vi "Configure Sequencer List ARB Cycles.vi"(7 "ARB Cycles (1)":i32=1, 8 "error in (no error)":errorcluster, 9 "Index (0)":i32, 10 "Instance (1)":i32=1, 11 "VISA resource name":refnum<visa-resource-name>) -> (0 "error out":errorcluster, 3 "VISA resource name out":refnum<visa-resource-name>)   [LabVIEW 2020, in "Rohde&Schwarz CMXP GPRF.lvlib"]
doc: "Defines the number of ARB cycles for the sequencer list entry with the selected Index.\n\nAttribute:\nRSCMXPGPRF_ATTR_SEQUENCER_LIST_ARB_CYCLES\n\nRemote-control command:\nSOURce:GPRF:GEN<i>:SEQuencer:LIST:ACYCles"
uses:
  <instrlib>/Rohde&Schwarz CMXP GPRF/Rohde&Schwarz CMXP GPRF.lvlib
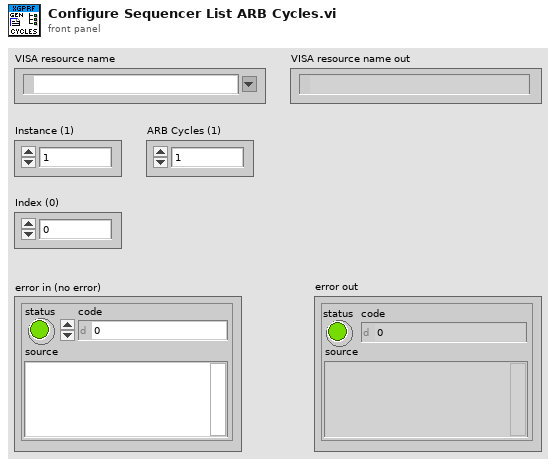
[diagram p1: front panel]
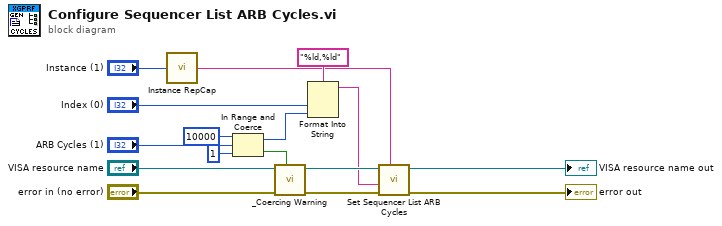
[diagram p0: block diagram]
diagram:
  n1 = call <instrlib>:"Instance RepCap.vi"("Instance in"="Instance (1)") -> ("Instance out"=w3:string)
  n2 = In Range and Coerce(upper limit=10000, x="ARB Cycles (1)", lower limit=1) -> (coerced(x)=w2:i32, In Range?=w10:bool)
  n3 = call <instrlib>:"_Coercing Warning.vi"("In Range?"=w10, "error in (no error)"="error in (no error)", "VISA resource name"="VISA resource name") -> ("error out"=w7:errorcluster, "VISA resource name out"=w6:refnum<visa-resource-name>)  [unwired: 7 in]
  n4 = Format Into String(format string="%ld,%ld", "Index (0)", w2) -> (resulting string=w1:string)  [unwired: 2 in, 1 out]
  n5 = call "Set Sequencer List ARB Cycles"("Repeated Capabilities"=w3, "error in (no error)"=w7, "Sequencer List ARB Cycles ()"=w1, "instrument handle"=w6) -> ("error out"=→"error out":errorcluster, "instrument handle out"=→"VISA resource name out":refnum<visa-resource-name>)  [unwired: 6 in]
